vi "Clean Up.vi"(8 "error in (no error)":errorcluster, 11 "Encoder Drive Straight in":refnum<class "Encoder Drive Straight.lvclass">) -> (0 "error out":errorcluster, 3 "Encoder Drive Straight out":refnum<class "Encoder Drive Straight.lvclass">)   [LabVIEW 2016, in "Encoder Drive Straight.lvclass"]
uses:
  Encoder Drive Straight.lvclass
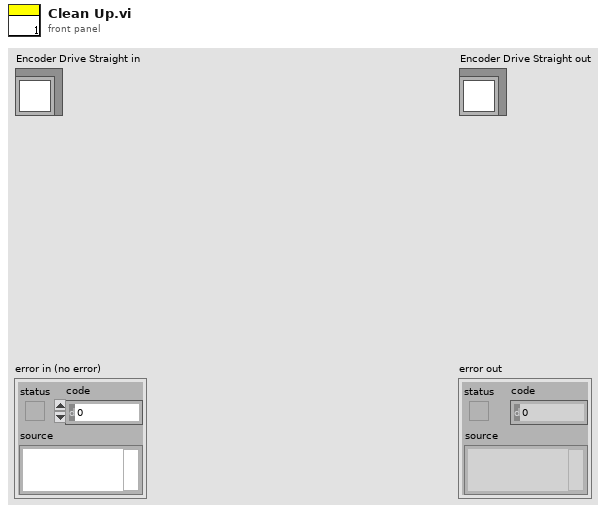
[diagram p1: front panel]
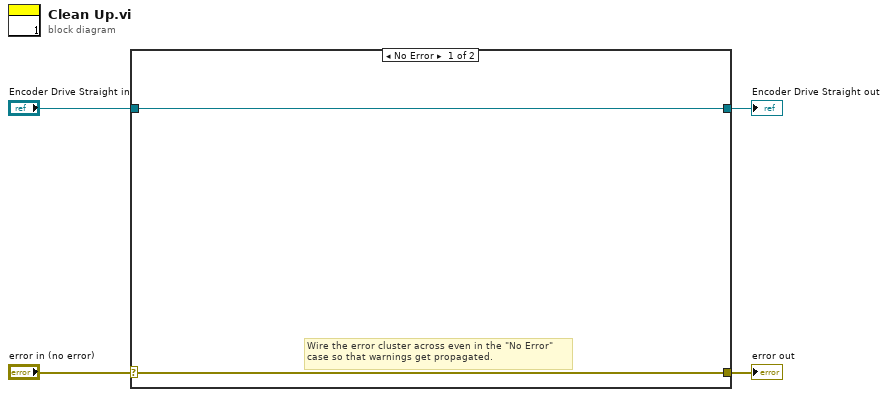
[diagram p0: block diagram]
diagram:
  n1 = case shown="No Error" "error in (no error)" {
    selector: "error in (no error)" -> [w5 w8]
    tunnel: [w5 w8] -> w3
    tunnel: [w6 w7] -> w1
    tunnel: "Encoder Drive Straight in" -> [w6 w7]
    frame No Error {
      # "Wire the error cluster across even in the \"No Error\"\ncase so that warnings get propagated."
    }
    frame Error {
    }
  }
  "error out" <- w3
  "Encoder Drive Straight out" <- w1
